vi "AddViews.vi"(8 "error in (no error)":errorcluster, 10 "Data":T1(array[cluster]), 11 "ViewMgr in":refnum<class "ViewMgr.lvclass">) -> (0 "error out":errorcluster, 3 "ViewMgr out":refnum<class "ViewMgr.lvclass">)   [LabVIEW 2020, in "CSM-TagDBDisplayContainer.lvlib" / "ViewMgr.lvclass"]
uses:
  ViewMgr.lvclass
  ViewMgr.lvclass/ViewMgr.ctl
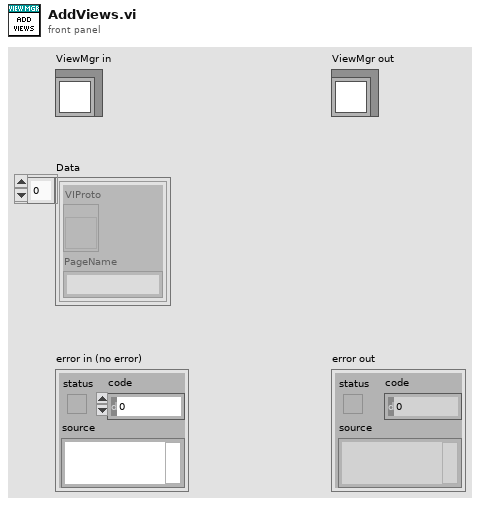
[diagram p1: front panel]
types:
  T1 = cluster{"VIProto":refnum<vi>, "PageName":string}[]
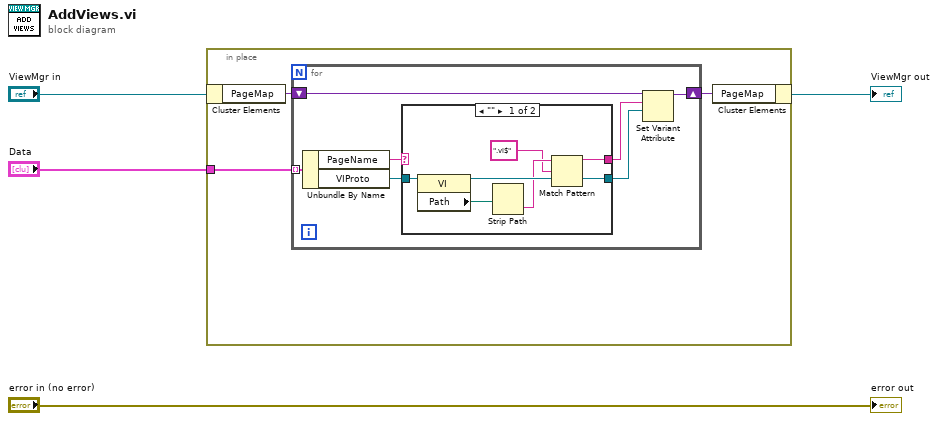
[diagram p0: block diagram]
diagram:
  n1 = in-place {
    in-place-border: "Data" -> [w5]
    n2 = in-place-cluster #1("ViewMgr in") -> ("PageMap"=w7:variant)
    n3 = for {
      shift-right: [w13] -> w6
      shift-left: w7 -> [w14]
      tunnel: w5 -> [w12] mode=indexing
      n4 = Unbundle By Name(w12) -> ("PageName"=w11:string, "VIProto"=w9:refnum<vi>)
      n5 = case shown="\"\"" w11 {
        selector: w11 -> [_ w21]
        tunnel: [w19 w22] -> w10
        tunnel: w9 -> [w20 w22]
        tunnel: [w16 w21] -> w8
        frame "" {
          n6 = property class="VI"(reference=w20) -> (reference out=w19:refnum<vi>, "Path"=w18:path)  [unwired: 1 in, 1 out]
          n7 = Strip Path(path=w18) -> (name=w17:string)  [unwired: 1 out]
          n8 = Match Pattern(string=w17, regular expression=".vi$" ("string")) -> (before substring=w16:string)  [unwired: 1 in, 3 out]
        }
        frame Default {
        }
      }
      n9 = Set Variant Attribute(Variant=w14, name=w8, value=w10) -> (Variant out=w13:variant)  [unwired: 1 in, 2 out]
    }
    n10 = in-place-cluster #1("PageMap"=w6) -> (→"ViewMgr out":refnum<class "ViewMgr.lvclass">)
  }
  "error out" <- "error in (no error)"
